vi "PID Advanced (DBL) Obsolete.vi"(0 "setpoint":dbl format="%.2f", 1 "output range":cluster{"output high":dbl, "output low":dbl}={"output high"=100.0, "output low"=-100.0} {"output low" format="%.2f"; "output high" format="%.2f"}, 2 "auto? (T)":bool=TRUE, 3 "manual control":dbl format="%.2f", 5 "process variable":dbl format="%.2f", 7 "setpoint range":cluster{"setpoint high":dbl, "setpoint low":dbl}={"setpoint high"=100.0, "setpoint low"=0.0} {"setpoint high" format="%.2f"; "setpoint low" format="%.2f"}, 9 "PID gains":T1={"proportional gain (Kc)"=1.0, "integral time (Ti, min)"=0.01, "derivative time (Td, min)"=0.0} {"derivative time (Td, min)" format="%.3f"; "integral time (Ti, min)" format="%.3f"; "proportional gain (Kc)" format="%.3f"}, 11 "dt (s)":dbl=-1.0 format="%.3f", 12 "reinitialize? (F)":bool, 13 "beta":dbl=1.0 format="%.2f", 14 "linearity":dbl=1.0 format="%.2f") -> (4 "output":dbl format="%.2f", 15 "dt out (s)":dbl format="%.3f")   [LabVIEW 2020, in "NI_PID_pid.lvlib"]
doc: "PID algorithm with advanced optional features. PID algorithm includes features of PID.vi as well as manual mode control with bumpless manual to automatic transitions, non-linear integral action, two degree of freedom control and error-squared control."
uses:
  NI_PID_pid.lvlib
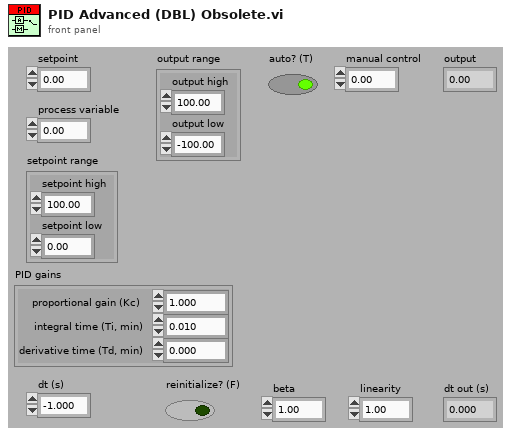
[diagram p1: front panel]
types:
  T1 = cluster{"proportional gain (Kc)":dbl, "integral time (Ti, min)":dbl, "derivative time (Td, min)":dbl}
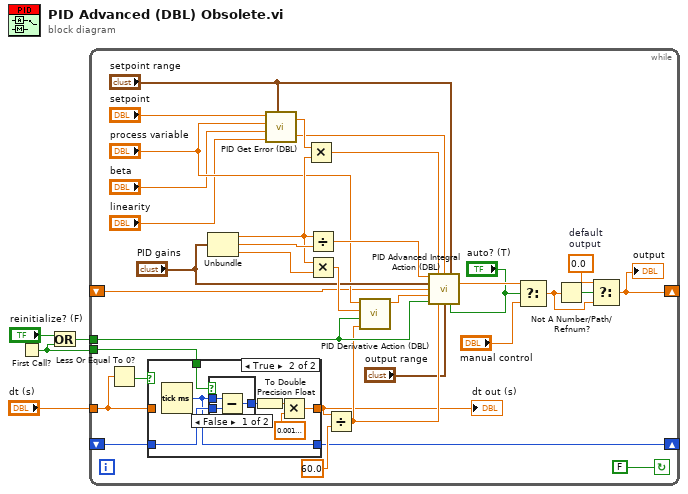
[diagram p0: block diagram]
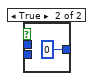
[diagram p3: hidden frame]
diagram:
  n1 = First Call?() -> (First Call?: T/F=w1:bool)
  n2 = Or(x="reinitialize? (F)", y=w1) -> (x .or. y?=w4:bool)
  n3 = while {
    shift-left: _ -> [w11]
    shift-right: [w16] -> _
    tunnel: w4 -> [w29]
    shift-left: _ -> [w8]
    shift-right: [w6] -> _
    tunnel: "dt (s)" -> [w9]
    tunnel: w1 -> [w5]
    stop <- FALSE continue-if-true
    w22 = 0.0  # default output
    n4 = Less Or Equal To 0?(x=w9) -> (x <= 0?=w10:bool)
    n5 = case shown="True" w10 {
      tunnel: [w40 w44] -> w7
      tunnel: w8 -> [w39 w43]
      tunnel: [w39 w42] -> w6
      tunnel: w9 -> [w40 _]
      tunnel: w5 -> [_ w41]
      frame False {
      }
      frame True {
        n6 = Tick Count (ms)() -> (millisecond timer value=w42:u32)
        n7 = case shown="False" w41 {
          tunnel: [w50 u32 0] -> w46
          tunnel: w43 -> [w49 _]
          tunnel: w42 -> [w48 _]
          frame False {
            n8 = Subtract(x=w48, y=w49) -> (x-y=w50:u32)
          }
          frame True {
          }
        }
        n9 = To Double Precision Float(number=w46) -> (double precision float=w45:dbl)
        n10 = Multiply(x=w45, y=0.0010000000474974513) -> (x*y=w44:dbl)
      }
    }
    "dt out (s)" <- w7
    n11 = Unbundle("PID gains") -> ("proportional gain (Kc)"=w34:dbl, "integral time (Ti, min)"=w37:dbl, "derivative time (Td, min)"=w36:dbl)
    n12 = call "PID Get Error (DBL).vi"("setpoint"="setpoint", "process variable"="process variable", "beta"="beta", "linearity"="linearity", "setpoint range"="setpoint range") -> ("error (with beta)"=w26:dbl, "error"=w15:dbl)
    n13 = Multiply(x=w26, y=w34) -> (x*y=w31:dbl)
    n14 = Divide(x=w34, y=w37) -> (x/y=w32:dbl)
    n15 = Multiply(x=w34, y=w36) -> (x*y=w35:dbl)
    n16 = Divide(x=w7, y=60.0) -> (x/y=w28:dbl)
    n17 = call "PID Derivative Action (DBL).vi"("dt (min)"=w28, "initialize (F)"=w29, "Kd"=w35, "process variable"="process variable") -> ("derivative action"=w30:dbl)  [unwired: 3 out]
    n18 = call "PID Advanced Integral Action (DBL).vi"("Ki"=w32, "proportional action"=w31, "error"=w15, "setpoint range"="setpoint range", "PID gains"="PID gains", "previous output"=w11, "derivative action"=w30, "initialize (F)"=w29, "dt (min)"=w28, "output range"="output range", "auto? (T)"="auto? (T)") -> ("output"=w20:dbl)  [unwired: 2 in, 2 out]
    n19 = Select(t=w20, s="auto? (T)", f="manual control") -> (s? t:f=w18:dbl)
    n20 = Not A Number/Path/Refnum?(number/path/refnum=w18) -> (NaN/Path/Refnum?=w21:bool)
    n21 = Select(t=w22, s=w21, f=w18) -> (s? t:f=w16:dbl)
    "output" <- w16
  }
